vi "Query Configuration Data.vi"(8 "error in (no error)":errorcluster, 11 "Ethernet in":refnum<class "ENET_BS1201.lvclass">) -> (0 "error out":errorcluster, 1 "Received":bool, 2 "Configuration Data":string, 3 "Ethernet out":refnum<class "ENET_BS1201.lvclass">)   [LabVIEW 2021, in "BS120x Driver.lvlib" / "ENET_BS1201.lvclass"]
uses:
  ENET_BS1201.lvclass
  C:/Users/Public/Documents/Projects/7100-00109 SW BS1201 LV Driver/trunk/source/ENET_BS120x/ENET_BS120x.lvclass
  ENET_BS120x/ENET_BS120x.lvclass
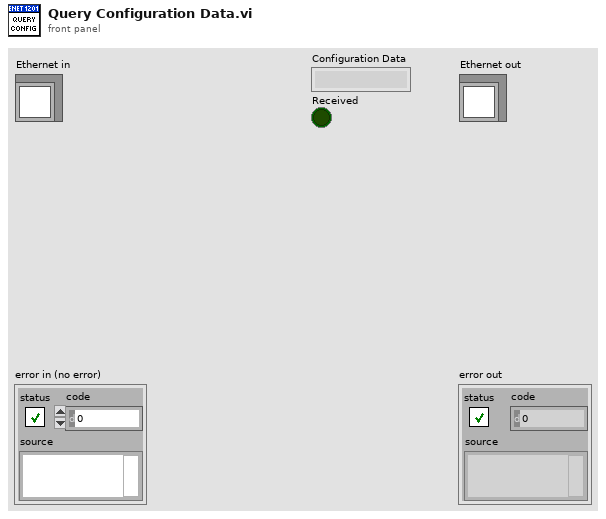
[diagram p1: front panel]
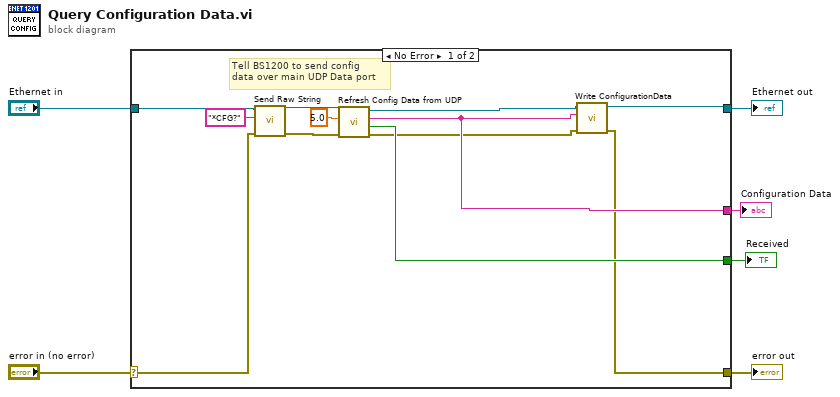
[diagram p0: block diagram]
diagram:
  n1 = case shown="No Error" "error in (no error)" {
    selector: "error in (no error)" -> [w13 w20]
    tunnel: [w7 w20] -> w5
    tunnel: [w10 w19] -> w3
    tunnel: "Ethernet in" -> [w16 w19]
    tunnel: [w9 _] -> w2
    tunnel: [w17 _] -> w1
    frame No Error {
      # "Tell BS1200 to send config\ndata over main UDP Data port"
      n2 = call "Send Raw String.vi"("error in (no error)"=w13, "String Data"="*CFG?", "ENET in"=w16) -> ("error out"=w12:errorcluster, "ENET out"=w14:refnum<class "ENET_BS1201.lvclass">)  [unwired: 7 in]
      n3 = call "Refresh Config Data from UDP.vi"("error in (no error)"=w12, "Timeout (2s)"=5.0, "Ethernet in"=w14) -> ("error out"=w8:errorcluster, "Received"=w17:bool, "Configuration Data"=w9:string, "Ethernet out"=w11:refnum<class "ENET_BS1201.lvclass">)  [unwired: 5 in]
      n4 = call-dynamic "Write ConfigurationData.vi"("error in (no error)"=w8, "ConfigurationData"=w9, "ENET_BS120x in"=w11) -> ("error out"=w7:errorcluster, "ENET_BS120x out"=w10:refnum<class "ENET_BS1201.lvclass">)  [unwired: 7 in]
    }
    frame Error {
    }
  }
  "error out" <- w5
  "Ethernet out" <- w3
  "Configuration Data" <- w2
  "Received" <- w1
